vi "Read Text File.vi"(8 "error in":errorcluster, 10 "offset (0)":i32, 11 "filepath":path=path "C:/Documents and Settings/user/Desktop/Claytons Archive/Calculate Statistics.vi") -> (0 "error out":errorcluster, 1 "size (bytes)":i64=-1, 2 "data":string)   [LabVIEW 2010]
doc: "This function opens an existing file, reads the entire file (as text), and closes the file.\n\nNote: This method is similar to the LabVIEW MD5 Checksum VI."
panel:
  # "File size is limited to 2 GB."
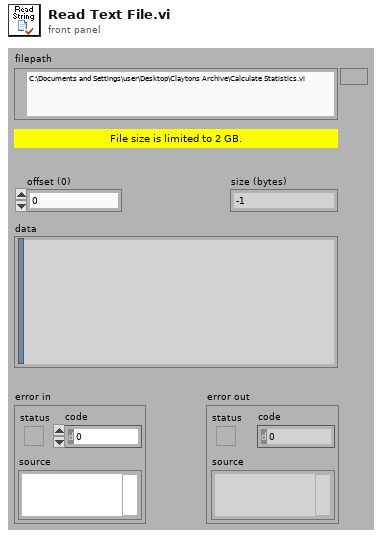
[diagram p1: front panel]
types:
  T1 = enum16{"open", "replace", "create", "open or create", "replace or create", "replace or create with confirmation"}
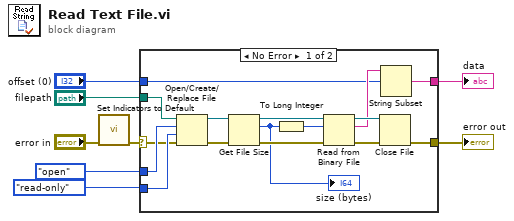
[diagram p0: block diagram]
diagram:
  n1 = call "Set Indicators to Default.vi"("error in"="error in") -> ("error out"=w2:errorcluster)  [unwired: 6 in]
  n2 = case shown="No Error" w2 {
    selector: w2 -> [w12 w25]
    tunnel: T1."open" ("operation (0:open)") -> [w24 _]
    tunnel: enum16{"read/write", "read-only", "write-only"}."read-only" ("access (0:read/write)") -> [w23 _]
    tunnel: "filepath" -> [w22 _]
    tunnel: [w10 _] -> w5
    tunnel: [w14 w25] -> w4
    tunnel: "offset (0)" -> [w9 _]
    frame No Error {
      n3 = Open/Create/Replace File(file path (use dialog)=w22, error in=w12, operation (0:open)=w24, access (0:read/write)=w23) -> (refnum out=w21:refnum<file>, error out=w19:errorcluster)  [unwired: 2 in, 1 out]
      n4 = Get File Size(file=w21, error in=w19) -> (refnum out=w20:refnum<file>, size (in bytes)=w16:i64, 0:w18:errorcluster)
      "size (bytes)" <- w16
      n5 = To Long Integer(number=w16) -> (32bit integer=w17:i32)
      n6 = Read from Binary File(8:w18, 10:w17, 11:w20) -> (0:w15:errorcluster, 2:w11:string, 3:w13:refnum<file>)  [unwired: 3 in, 1 out]
      n7 = Close File(refnum=w13, error in=w15) -> (error out=w14:errorcluster)  [unwired: 1 out]
      n8 = String Subset(string=w11, offset (0)=w9) -> (substring=w10:string)  [unwired: 1 in]
    }
    frame Error {
    }
  }
  "data" <- w5
  "error out" <- w4
